vi "Log.vi"(7 "Action":enum16{"None", "Write"}(ring), 8 "error in":errorcluster, 9 "Description":string, 10 "State":string, 11 "Page Name":string) -> (0 "error out":errorcluster)   [LabVIEW 2019]
uses:
  <vilib>/Utility/file.llb/Write Delimited Spreadsheet (string).vi
  Initialize/Initialize.lvlib
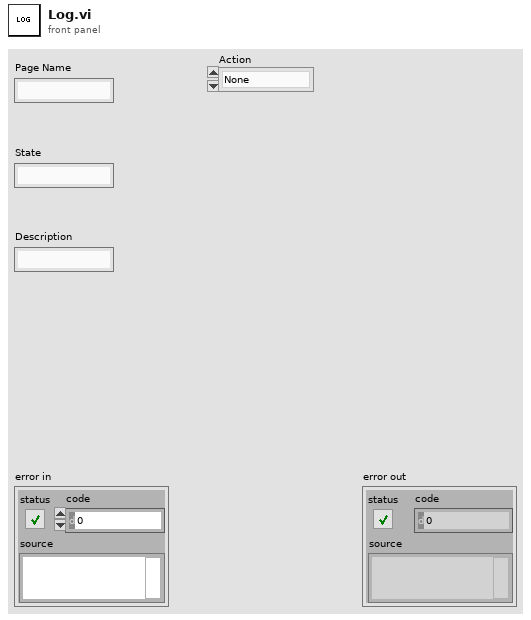
[diagram p1: front panel]
types:
  T1 = typedef "Initialize.lvlib/SEQ Data.ctl" = cluster{"Folder Path":path}
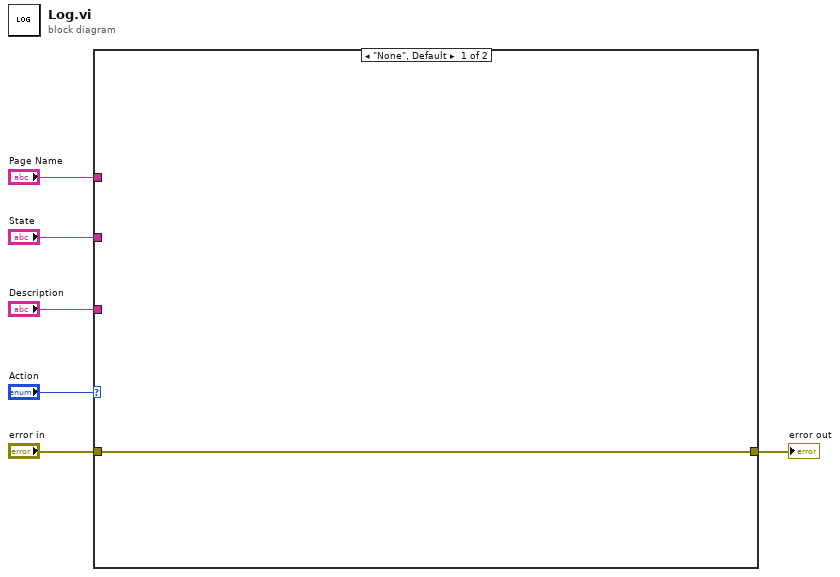
[diagram p0: block diagram]
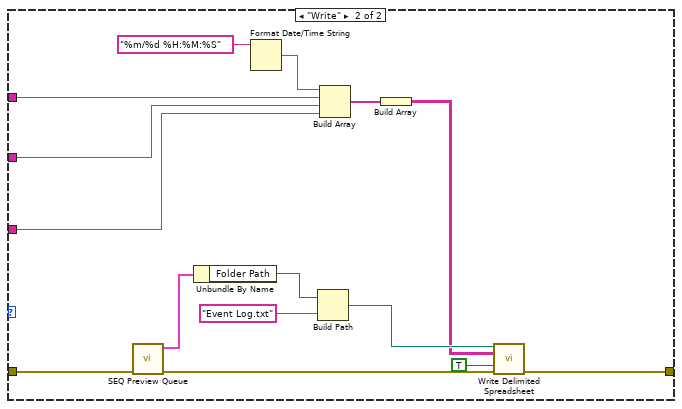
[diagram p2: hidden frame]
diagram:
  n1 = case shown="\"None\", Default" "Action" {
    tunnel: [w7 w19] -> w6
    tunnel: "Page Name" -> [_ w17]
    tunnel: "State" -> [_ w16]
    tunnel: "Description" -> [_ w15]
    tunnel: "error in" -> [w7 w8]
    frame "None", Default {
    }
    frame "Write" {
      n2 = call "SEQ Preview Queue.vi"("error in"=w8) -> ("error out"=w20:errorcluster, "SEQ Data"=w11:T1)  [unwired: 9 in]
      n3 = Unbundle By Name(w11) -> ("Folder Path"=w10:path)
      n4 = Format Date/Time String(time format string (%c)="%m/%d %H:%M:%S") -> (date/time string=w18:string)  [unwired: 2 in]
      n5 = Build Path(base path=w10, name or relative path="Event Log.txt") -> (appended path=w21:path)
      n6 = Build Array(w18, w17, w16, w15) -> (w14:string[])
      n7 = Build Array(w14) -> (w13:string[][])
      n8 = call-poly <vilib>:"Write Delimited Spreadsheet.vi"("file path (dialog if empty)"=w21, "2D data"=w13, "append to file? (new file:F)"=TRUE, "error in (no error)"=w20) -> ("error out"=w19:errorcluster)  [unwired: 10 in, 1 out]
    }
  }
  "error out" <- w6
